vi "Process data.vi"(8 "error in (no error)":errorcluster, 10 "input array":dbl[][](array[numeric]), 11 "ExampleClassDInverse in":refnum<class "ExampleClassDInverse.lvclass">) -> (0 "error out":errorcluster, 2 "output array":dbl[][](array[numeric]), 3 "ExampleClassDInverse out":refnum<class "ExampleClassDInverse.lvclass">)   [LabVIEW 2012, in "ExampleClassDInverse.lvclass"]
uses:
  ExampleClassDInverse.lvclass
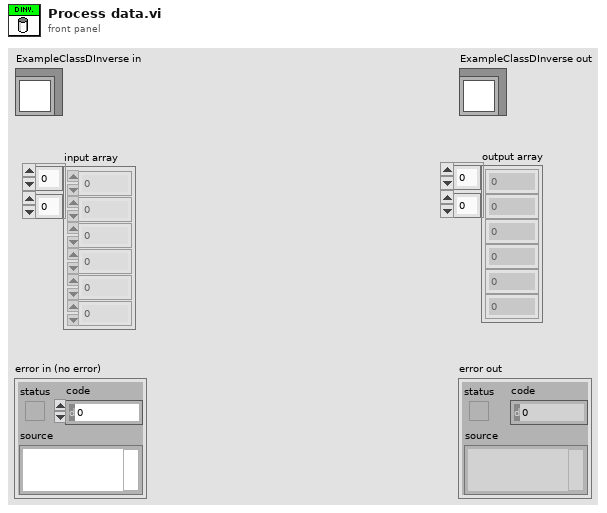
[diagram p1: front panel]
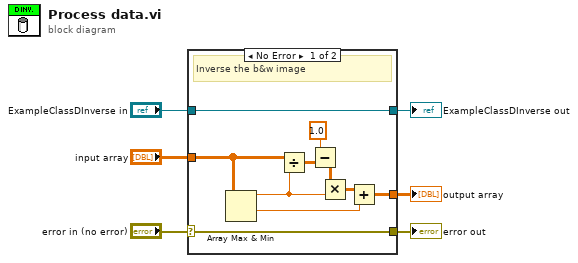
[diagram p0: block diagram]
diagram:
  n1 = case shown="No Error" "error in (no error)" {
    selector: "error in (no error)" -> [w10 w17]
    tunnel: "input array" -> [w12 w18]
    tunnel: [w7 w18] -> w5
    tunnel: [w11 w19] -> w3
    tunnel: "ExampleClassDInverse in" -> [w11 w19]
    tunnel: [w10 w17] -> w1
    frame No Error {
      # "Inverse the b&w image"
      n2 = Array Max & Min(array=w12) -> (max value=w13:dbl, min value=w9:dbl)  [unwired: 2 out]
      n3 = Divide(x=w12, y=w13) -> (x/y=w15:dbl[][])
      n4 = Subtract(x=1.0, y=w15) -> (x-y=w14:dbl[][])
      n5 = Multiply(x=w14, y=w13) -> (x*y=w8:dbl[][])
      n6 = Add(x=w8, y=w9) -> (x+y=w7:dbl[][])
    }
    frame Error {
    }
  }
  "error out" <- w1
  "ExampleClassDInverse out" <- w3
  "output array" <- w5
